vi "Initialize.vi"(8 "error in (no error)":errorcluster, 10 "ID Query (True)":bool=TRUE, 11 "VISA resource name":refnum<visa-resource-name>) -> (0 "error out":errorcluster, 3 "VISA resource name out":refnum<visa-resource-name>)   [LabVIEW 2024, in "Micron Optics sm130.lvlib"]
doc: "Establishes communication with the instrument and optionally performs an instrument identification query and/or an instrument reset. It also places the instrument in a default state needed for other instrument driver operations. Therefore, call this VI before calling other instrument driver VIs for this instrument. Generally, you need to call the Initialize VI only once at the beginning of an application."
uses:
  Micron Optics sm130.lvlib
panel:
  # "(c) 2009 - 2012 National Instruments.  ALL RIGHTS RESERVED."
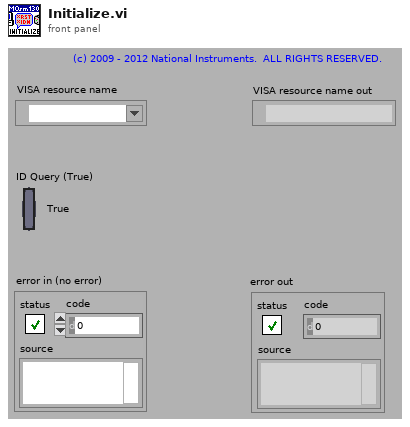
[diagram p1: front panel]
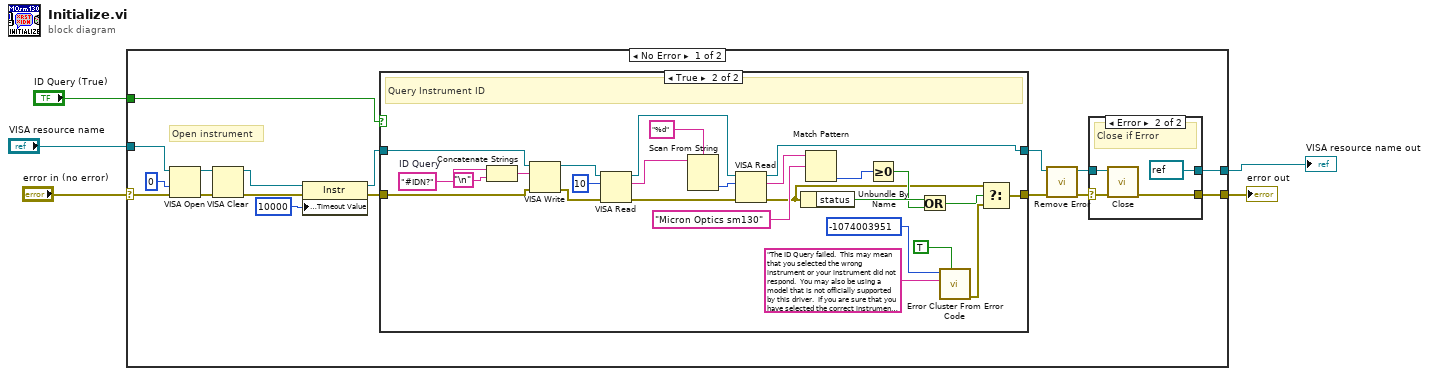
[diagram p0: block diagram]
diagram:
  n1 = case shown="No Error" "error in (no error)" {
    selector: "error in (no error)" -> [w6 w58]
    tunnel: "ID Query (True)" -> [w22 _]
    tunnel: "VISA resource name" -> [w21 w57]
    tunnel: [w14 w57] -> w3
    tunnel: [w13 w58] -> w2
    frame No Error {
      # "Open instrument"
      n2 = VISA Open(access mode=u32 0, error in (no error)=w6, VISA resource name=w21) -> (VISA resource name=w18:refnum<visa-resource-name>, error out=w17:errorcluster)  [unwired: 2 in]
      n3 = VISA Clear(VISA resource name=w18, error in (no error)=w17) -> (VISA resource name out=w16:refnum<visa-resource-name>, error out=w15:errorcluster)
      n4 = property class="Instr"(reference=w16, error in=w15, "General Settings:Timeout Value"=u32 10000) -> (reference out=w12:refnum<visa-resource-name>, error out=w11:errorcluster)
      n5 = case shown="True" w22 {
        tunnel: [w29 w56] -> w9
        tunnel: [w30 w39] -> w10
        tunnel: w12 -> [w30 w54]
        tunnel: w11 -> [w29 w55]
        frame False {
        }
        frame True {
          w33 = "#IDN?"  # ID Query
          # "Query Instrument ID"
          n6 = Concatenate Strings(w33, "\n") -> (w31:string)
          n7 = VISA Write(VISA resource name=w54, write buffer=w31, error in (no error)=w55) -> (VISA resource name out=w53:refnum<visa-resource-name>, error out=w52:errorcluster)  [unwired: 1 out]
          n8 = VISA Read(VISA resource name=w53, byte count=u32 10, error in (no error)=w52) -> (VISA resource name out=w41:refnum<visa-resource-name>, read buffer=w37:string, error out=w40:errorcluster)  [unwired: 1 out]
          n9 = Scan From String(format string="%d", input string=w37) -> (output 1=w36:i32)  [unwired: 3 in, 3 out]
          n10 = VISA Read(VISA resource name=w41, byte count=w36, error in (no error)=w40) -> (VISA resource name out=w39:refnum<visa-resource-name>, read buffer=w34:string, error out=w38:errorcluster)  [unwired: 1 out]
          n11 = Unbundle By Name(w38) -> ("status"=w44:bool)
          n12 = Match Pattern(string=w34, regular expression="Micron Optics sm130") -> (offset past match=w45:i32)  [unwired: 1 in, 3 out]
          n13 = Greater Or Equal To 0?(x=w45) -> (x >= 0?=w43:bool)
          n14 = Or(x=w44, y=w43) -> (x .or. y?=w42:bool)
          n15 = call <vilib>:"Error Cluster From Error Code.vi"("show call chain? (False)"=TRUE, "error message (\"\")"="The ID Query failed.  This may mean that you selected the wrong instrument or your instrument did not respond.  You may also be using a model that is not officially supported by this driver.  If you are sure that you have selected the correct instrument and it is responding, try disabling the ID Query." ("Source (VI Name)"), "error code (0)"=-1074003951 ("Code")) -> ("error out"=w49:errorcluster)  [unwired: 6 in]
          n16 = Select(t=w38, s=w42, f=w49) -> (s? t:f=w56:errorcluster)
        }
      }
      n17 = call "Remove Error.vi"("error in (no error)"=w9, "VISA resource name"=w10) -> ("error out"=w7:errorcluster, "VISA resource name out"=w8:refnum<visa-resource-name>)  [unwired: 8 in]
      n18 = case shown="Error" w7 {
        selector: w7 -> [w23 w26]
        tunnel: w8 -> [w24 w27]
        tunnel: [w24 refnum<visa-resource-name> refnum ("VISA resource name out")] -> w14
        tunnel: [w23 w28] -> w13
        frame No Error {
        }
        frame Error {
          # "Close if Error"
          n19 = call "Close.vi"("error in (no error)"=w26, "VISA resource name"=w27) -> ("error out"=w28:errorcluster)  [unwired: 9 in]
        }
      }
    }
    frame Error {
    }
  }
  "VISA resource name out" <- w3
  "error out" <- w2
